vi "Set Column Width.vi"(7 "AutoSizeMode":i32(ring)=1 items=["None"=1, "ColumnHeader"=2, "AllCellsExceptHeader"=4, "AllCells"=6, "DisplayedCellsExceptHeader"=8, "DisplayedCells"=10, "Fill"=16], 9 "FillWeight":sgl, 10 "MinWidth":u32, 11 "Column Descriptor in":T1={"name"="Link", "caption"="", "Column Type"=enum."String", "Params"="", "AutoSizeMode"=1, "FillWeight"=100.0, "MinWidth"=50, "tooltip"="The quick brown fox jumps over the lazy dog", "Enum Reference"=refnum, "Channel suffix"="", "Read Only"=FALSE, "Call Back VI"=refnum, "DT Dependency"=0, "name dependency"=0, "data type"=enum."Double", "Custom Column"=refnum} {"MinWidth" min=2 step=1; "AutoSizeMode" items=["None"=1, "ColumnHeader"=2, "AllCellsExceptHeader"=4, "AllCells"=6, "DisplayedCellsExceptHeader"=8, "DisplayedCells"=10, "Fill"=16]; "FillWeight" min=1 max=100}) -> (3 "Column Descriptor out":T1={"name"="Link", "caption"="", "Column Type"=enum."String", "Params"="", "AutoSizeMode"=1, "FillWeight"=100.0, "MinWidth"=50, "tooltip"="The quick brown fox jumps over the lazy dog", "Enum Reference"=refnum, "Channel suffix"="", "Read Only"=FALSE, "Call Back VI"=refnum, "DT Dependency"=0, "name dependency"=0, "data type"=enum."Double", "Custom Column"=refnum} {"MinWidth" min=2 step=1; "AutoSizeMode" items=["None"=1, "ColumnHeader"=2, "AllCellsExceptHeader"=4, "AllCells"=6, "DisplayedCellsExceptHeader"=8, "DisplayedCells"=10, "Fill"=16]; "FillWeight" min=1 max=100})   [LabVIEW 2013, in "Table Manager.lvlib" / "Column.lvclass"]
doc: "Sets the 'MinWidth', 'AutoSizeMode', and 'FillWeight' of a column."
uses:
  Column.lvclass
  Column Descriptor.ctl
  Column Type.ctl
  <vilib>/NI/Tag Bus/tag/Data Type.ctl
  Table Manager/Call Back Ref Type Def.ctl
  Configuration Editor/Classes/Engine Parent/Engine Parent Editor Node.lvclass
  Configuration Editor/Classes/Module editor node/module editor node.lvclass
  <vilib>/NI/Tag Bus/tag/tag descriptor.lvclass
  Table Manager/Table Manager.lvclass
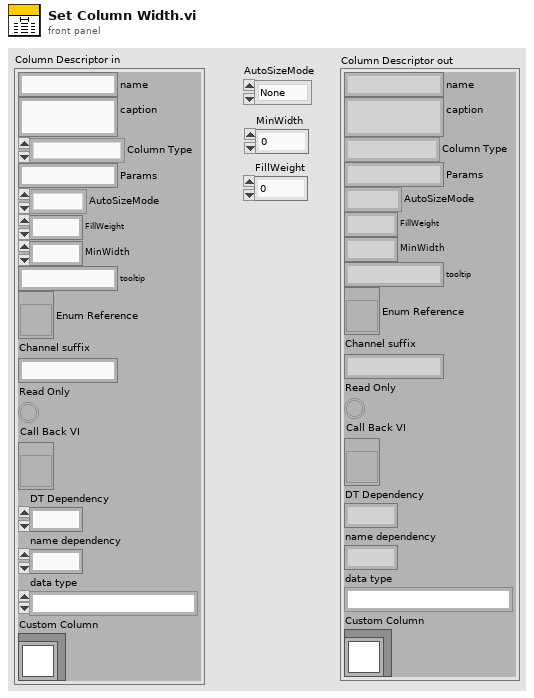
[diagram p1: front panel]
types:
  T1 = typedef "Table Manager.lvlib/Column.lvclass/Column Descriptor.ctl" = cluster{"name":string, "caption":string, "Column Type":T2, "Params":string, "AutoSizeMode":i32, "FillWeight":sgl, "MinWidth":u32, "tooltip":string, "Enum Reference":refnum<vi>, "Channel suffix":string, "Read Only":bool, "Call Back VI":T3, "DT Dependency":i32, "name dependency":i32, "data type":T4, "Custom Column":refnum<class "Column.lvclass">}
  T2 = typedef "Table Manager.lvlib/Column.lvclass/Column Type.ctl" = enum16{"String", "Mapping", "Enum", "Custom"}
  T3 = typedef "Table Manager.lvlib/Table Manager.lvclass/Call Back Ref Type Def.ctl" = refnum<vi>
  T4 = typedef "tag bus.lvlib/tag descriptor.lvclass/Data Type.ctl" = enum16{"Double", "Single", "I64", "I32", "I16", "I8", "U64", "U32", "U16", "U8", "Boolean", "String", "Array of Double", "Array of Single", "Array of I64", "Array of I32", "Array of I16", "Array of I8", "Array of U64", "Array of U32", "Array of U16", "Array of U8", "Array of Boolean", "Array of String"}
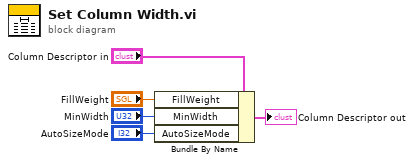
[diagram p0: block diagram]
diagram:
  n1 = Bundle By Name(cluster="Column Descriptor in", "FillWeight"="FillWeight", "MinWidth"="MinWidth", "AutoSizeMode"="AutoSizeMode") -> (→"Column Descriptor out":T1)
